vi "LED_with_wait.vi"(7 "FPGA I/O In":refnum<k21>="IO Module\\D0 0", 8 "Testpulse Time Delay (20 ns ticks)":u32=15, 9 "Testpulse Separation (20 ns ticks)":u32=500, 10 "Testpulse duration (20 ns ticks)":u32=1, 11 "Testpulser On/Off":bool) -> (0 "Total number of pulses sent":u64, 3 "Is Test Pulse?":bool)   [LabVIEW 2012]
uses:
  <vilib>/rvi/eio/common/nirviEmuTemplateMethod_errors.vi
  <vilib>/eio/EIONode/EIONode.xnode
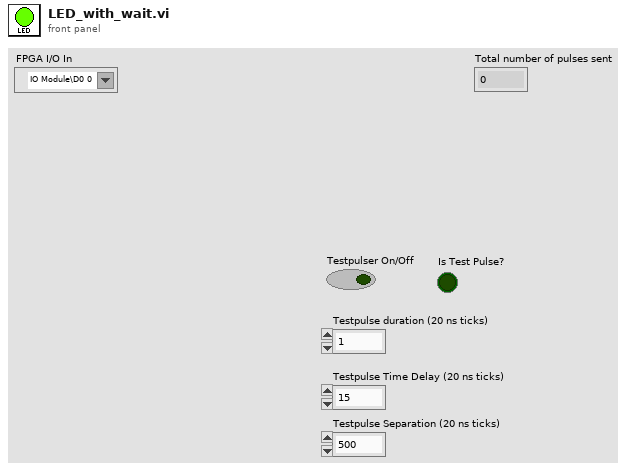
[diagram p1: front panel]
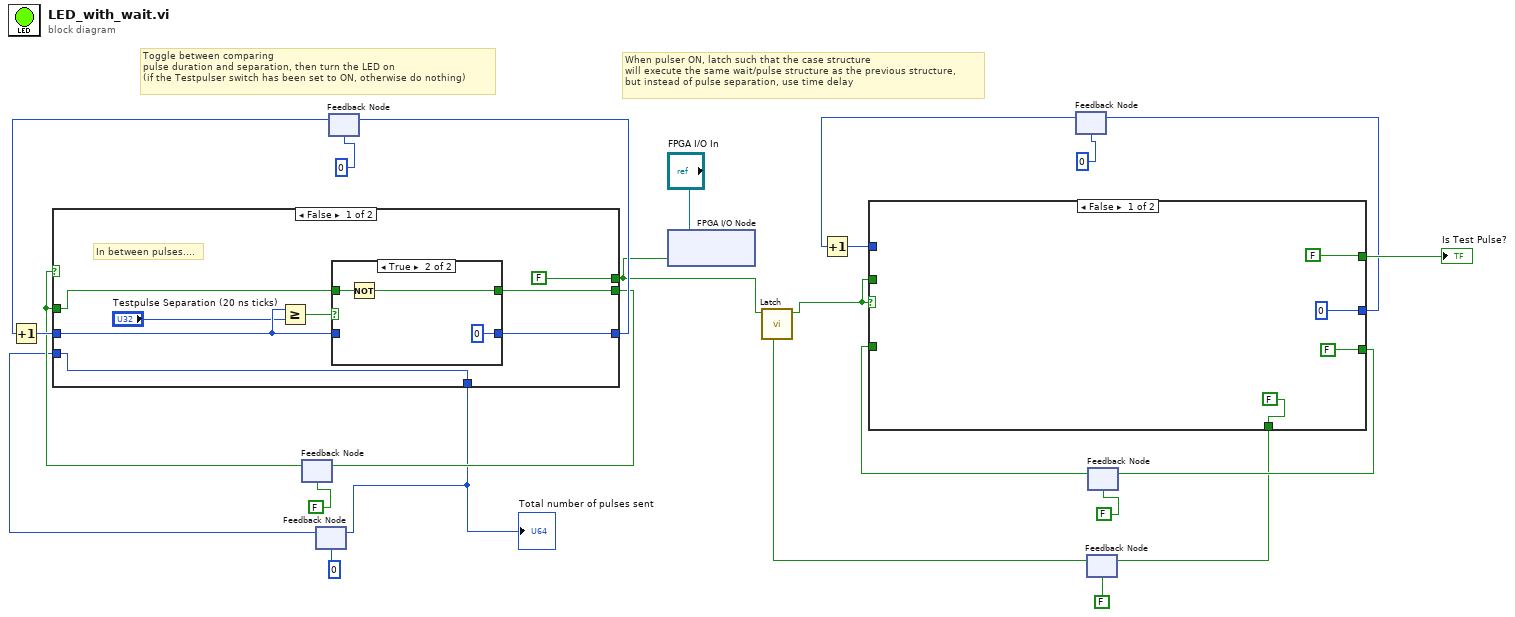
[diagram p0: block diagram]
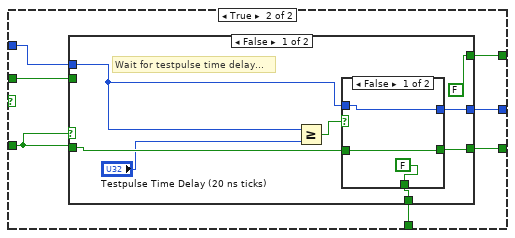
[diagram p2: hidden frame]
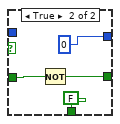
[diagram p3: hidden frame]
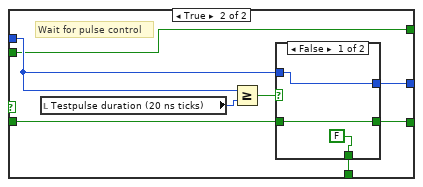
[diagram p4: hidden frame]
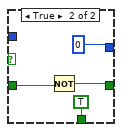
[diagram p5: hidden frame]
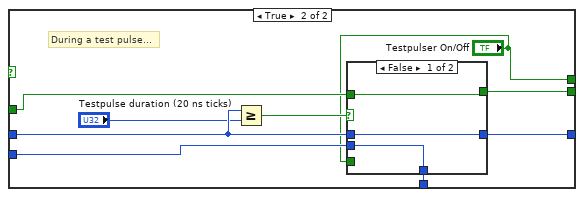
[diagram p7: hidden frame]
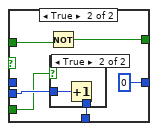
[diagram p8: hidden frame]
diagram:
  # "Toggle between comparing \npulse duration and separation, then turn the LED on\n(if the Testpulser switch has been set to ON, otherwise do nothing)"
  # "When pulser ON, latch such that the case structure\nwill execute the same wait/pulse structure as the previous structure, \nbut instead of pulse separation, use time delay"
  n1 = feedback #1(FALSE) -> (w18:bool)
  n2 = feedback #2(u64 0) -> (w2:u64)
  n3 = feedback #3(u32 0) -> (w21:u32)
  n4 = Increment(x=w21) -> (x+1=w24:u32)
  n5 = case shown="False" w18 {
    tunnel: w24 -> [w29 w44]
    tunnel: [w32 w45] -> w20
    tunnel: [w31 w46] -> w10
    tunnel: [FALSE ("IO Module\\D0 0") "Testpulser On/Off"] -> w5
    tunnel: w18 -> [w26 w41]
    tunnel: w2 -> [w25 w40]
    tunnel: [w25 w39] -> w3
    frame False {
      # "In between pulses...."
      n6 = Greater Or Equal?(x=w29, y="Testpulse Separation (20 ns ticks)") -> (x >= y?=w28:bool)
      n7 = case shown="True" w28 {
        tunnel: [w34 u32 0] -> w32
        tunnel: w29 -> [w34 _]
        tunnel: [w33 w36] -> w31
        tunnel: w26 -> [w33 w35]
        frame False {
        }
        frame True {
          n8 = Not(x=w35) -> (.not. x?=w36:bool)
        }
      }
    }
    frame True {
      # "During a test pulse..."
      n9 = Greater Or Equal?(x=w44, y="Testpulse duration (20 ns ticks)") -> (x >= y?=w43:bool)
      n10 = case shown="False" w43 {
        tunnel: w44 -> [w49 _]
        tunnel: [w48 w55] -> w46
        tunnel: [w49 u32 0] -> w45
        tunnel: w41 -> [w48 w53]
        tunnel: w40 -> [w47 w52]
        tunnel: [w47 w51] -> w39
        tunnel: "Testpulser On/Off" -> [_ w50]
        frame False {
        }
        frame True {
          n11 = Not(x=w53) -> (.not. x?=w55:bool)
          n12 = case shown="True" w50 {
            tunnel: w52 -> [w56 w58]
            tunnel: [w56 w57] -> w51
            frame False {
            }
            frame True {
              n13 = Increment(x=w58) -> (x+1=w57:u64)
            }
          }
        }
      }
    }
  }
  "Total number of pulses sent" <- w3
  n14 = feedback-in #1(w10) -> ()
  n15 = feedback-in #2(w3) -> ()
  n16 = feedback-in #3(w20) -> ()
  n17 = xnode "FPGA I/O Node"("I/O Item"=w5, "FPGA I/O In"="FPGA I/O In") -> ()  [unwired: 1 out]
  n18 = feedback #4(u32 0) -> (w16:u32)
  n19 = Increment(x=w16) -> (x+1=w15:u32)
  n20 = feedback #5(FALSE) -> (w7:bool)
  n21 = call "Latch.vi"("Reset"=w7, "Input"=w5) -> ("Output"=w6:bool)  [unwired: 9 in]
  n22 = feedback #6(FALSE) -> (w12:bool)
  n23 = case shown="False" w6 {
    tunnel: w6 -> [_ w64]
    tunnel: [FALSE w66] -> w23
    tunnel: w15 -> [_ w67]
    tunnel: [u32 0 w65] -> w14
    tunnel: w12 -> [_ w69]
    tunnel: [FALSE w68] -> w11
    tunnel: [FALSE w63] -> w8
    frame False {
    }
    frame True {
      n24 = case shown="False" w69 {
        tunnel: w69 -> [w76 w89]
        tunnel: [w75 w88] -> w68
        tunnel: w67 -> [w72 w90]
        tunnel: [FALSE w86] -> w66
        tunnel: [w73 w87] -> w65
        tunnel: w64 -> [_ w86]
        tunnel: [w70 w85] -> w63
        frame False {
          # "Wait for testpulse time delay..."
          n25 = Greater Or Equal?(x=w72, y="Testpulse Time Delay (20 ns ticks)") -> (x >= y?=w77:bool)
          n26 = case shown="False" w77 {
            tunnel: w76 -> [w80 w84]
            tunnel: [w80 w83] -> w75
            tunnel: [w79 u32 0] -> w73
            tunnel: w72 -> [w79 _]
            tunnel: [FALSE FALSE] -> w70
            frame False {
            }
            frame True {
              n27 = Not(x=w84) -> (.not. x?=w83:bool)
            }
          }
        }
        frame True {
          # "Wait for pulse control"
          n28 = local read "Testpulse duration (20 ns ticks)"() -> (w92:u32)
          n29 = Greater Or Equal?(x=w90, y=w92) -> (x >= y?=w91:bool)
          n30 = case shown="False" w91 {
            tunnel: w90 -> [w94 _]
            tunnel: w89 -> [w95 w98]
            tunnel: [w95 w97] -> w88
            tunnel: [w94 u32 0] -> w87
            tunnel: [FALSE TRUE] -> w85
            frame False {
            }
            frame True {
              n31 = Not(x=w98) -> (.not. x?=w97:bool)
            }
          }
        }
      }
    }
  }
  "Is Test Pulse?" <- w23
  n32 = feedback-in #4(w14) -> ()
  n33 = feedback-in #5(w8) -> ()
  n34 = feedback-in #6(w11) -> ()
